vi "Latihan 6 (For Loop).vi"() -> ()   [LabVIEW 2021]
uses:
  <vilib>/numeric/Random Number (Range) U64.vi
  <vilib>/numeric/sub_Random U32.vi
panel:
  out "Numeric 2":dbl
  out "Numeric":dbl
  out "Array 2":dbl[](array[numeric])
  out "Array":dbl[](array[numeric])
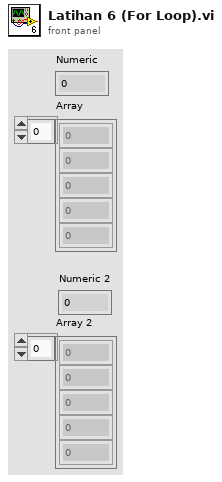
[diagram p1: front panel]
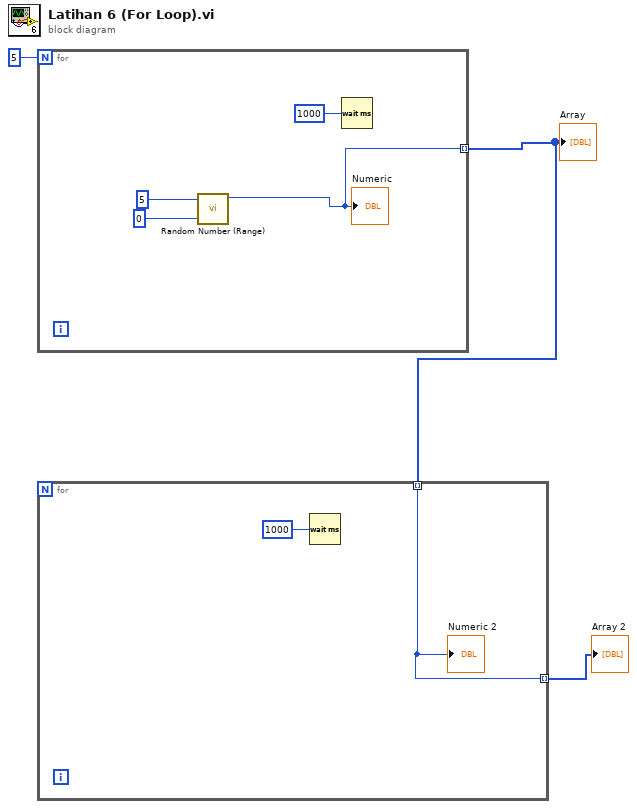
[diagram p0: block diagram]
diagram:
  n1 = for {
    N: 5 -> [_]
    tunnel: [w4] -> w2 mode=indexing
    n2 = call-poly <vilib>:"Random Number (Range).vi"("lower bound (0)"=u64 0, "upper bound (100)"=u64 5) -> ("number"=w4:u64)  [unwired: 9 in]
    "Numeric" <- w4
    n3 = Wait (ms)(milliseconds to wait=u32 1000) -> ()  [unwired: 1 out]
  }
  "Array" <- w2
  n4 = for {
    tunnel: w2 -> [w8] mode=indexing
    tunnel: [w8] -> w1 mode=indexing
    n5 = Wait (ms)(milliseconds to wait=u32 1000) -> ()  [unwired: 1 out]
    "Numeric 2" <- w8
  }
  "Array 2" <- w1
